vi "TCP Connection FGV.vi"(6 "timeout ms (20000)":i32=20000, 7 "MQTT Broker":cluster{"address (IP)":string, "port":u16}={"address (IP)"="broker.mqttdashboard.com", "port"=1883}, 8 "error in":errorcluster, 10 "Command":T1) -> (0 "error out":errorcluster, 3 "Connection ID":refnum<k5>)   [LabVIEW 2020, in "DAQIO MQTT.lvlib"]
uses:
  DAQIO MQTT.lvlib
  Controls/Connection FGV Actions.ctl
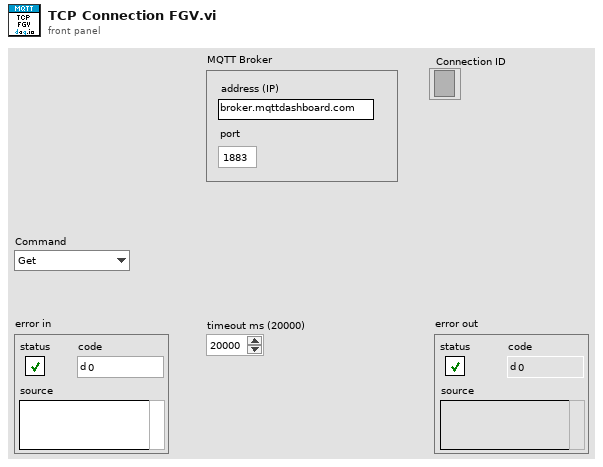
[diagram p1: front panel]
types:
  T1 = typedef "DAQIO MQTT.lvlib/Connection FGV Actions.ctl" = enum16{"Get", "Set", "Delete"}
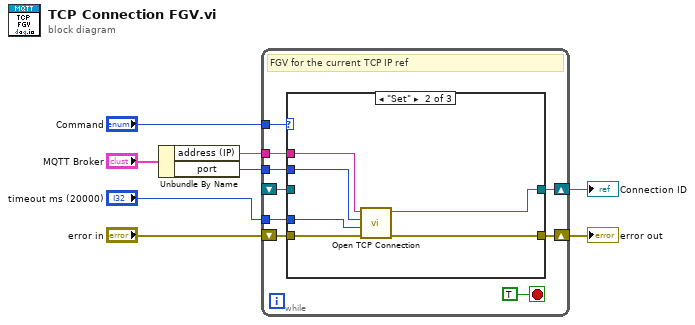
[diagram p0: block diagram]
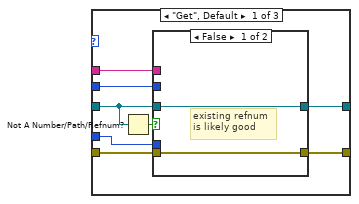
[diagram p2: hidden frame]
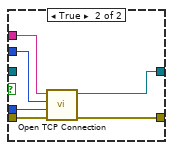
[diagram p3: hidden frame]
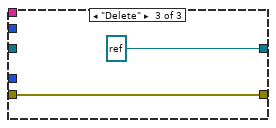
[diagram p4: hidden frame]
diagram:
  n1 = Unbundle By Name("MQTT Broker") -> ("address (IP)"=w2:string, "port"=w1:u16)
  n2 = while {
    shift-right: [w15] -> w6
    shift-left: "error in" -> [w16]
    shift-right: [w14] -> w8
    shift-left: _ -> [w13]
    tunnel: "timeout ms (20000)" -> [w12]
    tunnel: "Command" -> [w11]
    tunnel: w2 -> [w10]
    tunnel: w1 -> [w9]
    stop <- TRUE stop-if-true
    # "FGV for the current TCP IP ref"
    n3 = case shown="\"Set\"" w11 {
      tunnel: w10 -> [w24 w39 _]
      tunnel: w9 -> [w23 w38 _]
      tunnel: w16 -> [w21 w37 w40]
      tunnel: [w20 w36 w40] -> w15
      tunnel: [w19 w35 refnum<k5> refnum ("connection ID")] -> w14
      tunnel: w13 -> [w18 _ _]
      tunnel: w12 -> [w22 w34 _]
      frame "Get", Default {
        n4 = Not A Number/Path/Refnum?(number/path/refnum=w18) -> (NaN/Path/Refnum?=w25:bool)
        n5 = case shown="False" w25 {
          tunnel: w24 -> [_ w33]
          tunnel: w23 -> [_ w32]
          tunnel: w22 -> [_ w31]
          tunnel: w21 -> [w26 w30]
          tunnel: [w26 w29] -> w20
          tunnel: [w27 w28] -> w19
          tunnel: w18 -> [w27 _]
          frame False {
            # "existing refnum\nis likely good"
          }
          frame True {
            n6 = call "Open TCP Connection.vi"("error in (no error)"=w30, "timeout ms (20000)"=w31, "remote port or service name"=w32, "address"=w33) -> ("error out"=w29:errorcluster, "connection ID"=w28:refnum<k5>)  [unwired: 6 in]
          }
        }
      }
      frame "Set" {
        n7 = call "Open TCP Connection.vi"("error in (no error)"=w37, "timeout ms (20000)"=w34, "remote port or service name"=w38, "address"=w39) -> ("error out"=w36:errorcluster, "connection ID"=w35:refnum<k5>)  [unwired: 6 in]
      }
      frame "Delete" {
      }
    }
  }
  "Connection ID" <- w8
  "error out" <- w6
